vi "ZPL Wait ms.vi"(8 "error":errorcluster, 10 "Delay (1 mS)":u32=1, 11 "VISA":refnum<visa-resource-name>) -> (0 "error out":errorcluster, 3 "VISA out":refnum<visa-resource-name>)   [LabVIEW 2016]
doc: "Wait number of milliseconds. Used for allowing instrument to settle after changing the output. If \"Delay\" input not wired, it will wait 1 mSec.\n\nIf \"error\" input is set to error, the VI will not wait."
panel:
  # "Lambda ZPLUS \n Serial Port\n  DC Power Supplies"
  # "WAIT\nmilliseconds"
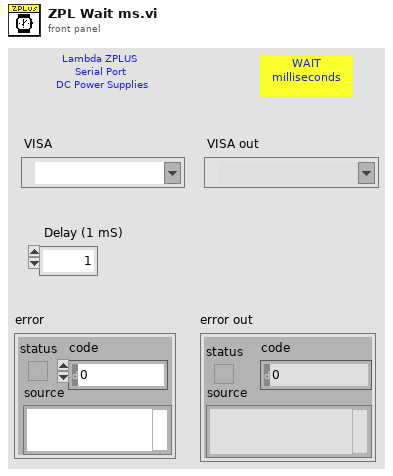
[diagram p1: front panel]
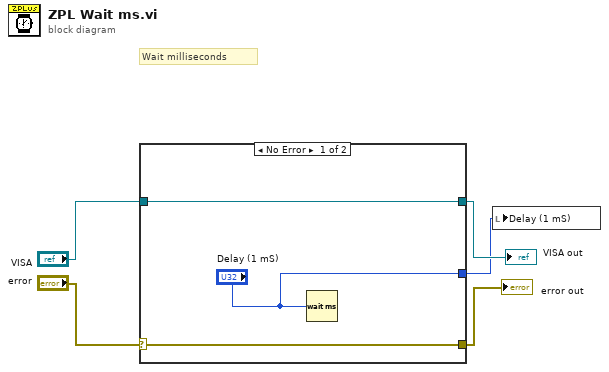
[diagram p0: block diagram]
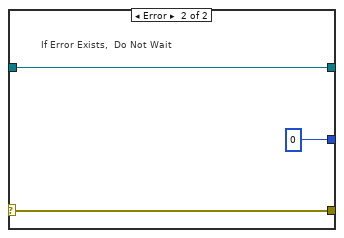
[diagram p2: hidden frame]
diagram:
  # "Wait milliseconds"
  n1 = case shown="No Error" "error" {
    selector: "error" -> [w8 w10]
    tunnel: [w8 w10] -> w2
    tunnel: "VISA" -> [w7 w11]
    tunnel: [w7 w11] -> w3
    tunnel: ["Delay (1 mS)" u32 0 ("Delay (20 mS)")] -> w1
    frame No Error {
      n2 = Wait (ms)(milliseconds to wait="Delay (1 mS)") -> ()  [unwired: 1 out]
    }
    frame Error {
      # "If Error Exists,  Do Not Wait"
    }
  }
  "error out" <- w2
  "VISA out" <- w3
  n3 = local write "Delay (1 mS)"(w1) -> ()
